vi "errinfo.vi"(1 "VCI_ERR_INFO":T1) -> ()   [LabVIEW 2020]
panel:
  out "ArLost_ErrData":u8
  out "Passive_ErrData2":u8
  out "Passive_ErrData1":u8
  out "Passive_ErrData0":u8
  out "ErrCode":u32
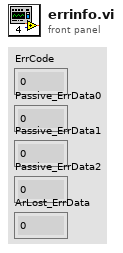
[diagram p1: front panel]
types:
  T1 = cluster{"ErrCode":u32, "Passive_ErrData0":u8, "Passive_ErrData1":u8, "Passive_ErrData2":u8, "ArLost_ErrData":u8}
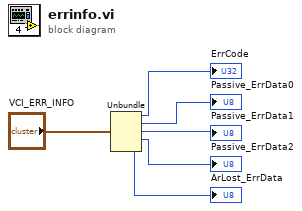
[diagram p0: block diagram]
diagram:
  n1 = Unbundle("VCI_ERR_INFO") -> ("ErrCode"=→"ErrCode":u32, "Passive_ErrData0"=→"Passive_ErrData0":u8, "Passive_ErrData1"=→"Passive_ErrData1":u8, "Passive_ErrData2"=→"Passive_ErrData2":u8, "ArLost_ErrData"=→"ArLost_ErrData":u8)
